vi "Detach Servo.vi"(0 "Arduino Resource":T1={"VISA resource"="", "Board Type"=enum."Arduino Uno", "Connection Type"=enum."USB / Serial", "Bytes Per Packet (15)"=15}, 5 "Servo Number":u8, 11 "error in":errorcluster) -> (4 "Arduino Resource":T1={"VISA resource"="", "Board Type"=enum."Arduino Uno", "Connection Type"=enum."USB / Serial", "Bytes Per Packet (15)"=15}, 15 "error out":errorcluster)   [LabVIEW 2011, in "LabVIEW Interface for Arduino.lvlib"]
doc: "Detach Servo release the servo from its assigned pin allowing you to use the DIO pin for general purpose digital input and output."
uses:
  <vilib>/LabVIEW Interface for Arduino/LabVIEW Interface for Arduino.lvlib
  <vilib>/LabVIEW Interface for Arduino/Private/Type Defs/Arduino Resource.ctl
  <vilib>/LabVIEW Interface for Arduino/Private/Type Defs/Board Type.ctl
  <vilib>/LabVIEW Interface for Arduino/Private/Type Defs/Command.ctl
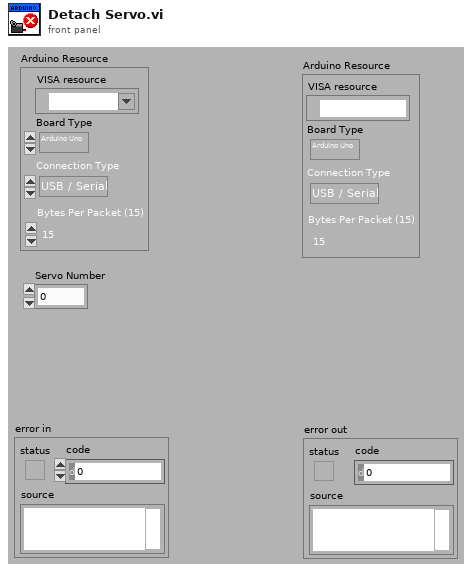
[diagram p1: front panel]
types:
  T1 = typedef "LabVIEW Interface for Arduino.lvlib/Arduino Resource.ctl" = cluster{"VISA resource":refnum<visa-resource-name>, "Board Type":T2, "Connection Type":enum8{"USB / Serial"}, "Bytes Per Packet (15)":u8}
  T2 = typedef "LabVIEW Interface for Arduino.lvlib/Board Type.ctl" = enum16{"Arduino Uno", "Dimuelanove w/Atmega 328", "Mega 2560", "Chipkit Uno32", "Chipkit Max32"}
  T3 = typedef "LabVIEW Interface for Arduino.lvlib/Command.ctl" = enum8{"setArduinoMode", "flushSerial", "setPinMode", "digitalWritePin", "digitalWritePort", "tone", "digitalReadPin", "digitalReadPort", "analogReadPin", "analogReadPort", "pwmWritePin", "pwmWritePort", "sevenSegment_Configure", "sevenSegment_Write", "I2C Init", "I2C Write", "I2C Read", "SPI Init", "SPI Set Bit Order", "SPI Set Clock Divider", "SPI Set Data Mode", "SPI Send / Receive", "SPI Close", "Servo Set Num Servos", "Servo Config Servo", "Servo Write Angle", "Servo Read Angle", "Servo Write Pulse Width", "Servo Read Pulse Width", "Servo Detach", "LCD Init", "LCD Set Size", "LCD Set Cursor Mode", "LCD Clear", "LCD Set Cursor Position", "LCD Print", "LCD Display Power", "LCD Scroll Display", "LCD Autoscroll", "LCD Print Direction", "LCD Create Custom Char", "LCD Print Custom Char", "contAcqOn", "contAcqOff", "getFirmwareVersion", "FiniteSampleStart"}
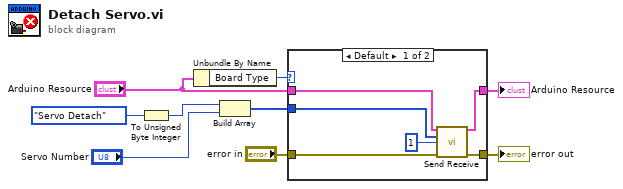
[diagram p0: block diagram]
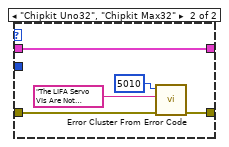
[diagram p2: hidden frame]
diagram:
  n1 = To Unsigned Byte Integer(number=Command."Servo Detach" ("Command")) -> (unsigned 8bit integer=w8:u8)
  n2 = Unbundle By Name("Arduino Resource") -> ("Board Type"=w2:T2)
  n3 = Build Array(w8, "Servo Number") -> (w6:u8[])
  n4 = case shown="Default" w2 {
    tunnel: "error in" -> [w14 w18]
    tunnel: [w11 w17] -> w4
    tunnel: "Arduino Resource" -> [w13 w16]
    tunnel: [w12 w16] -> w5
    tunnel: w6 -> [w10 _]
    frame Default {
      n5 = call <vilib>:"Send Receive.vi"("Arduino Resource"=w13, "Data"=w10, "Bytes To Read (0)"=u8 1, "error in"=w14) -> ("Arduino Resource"=w12:T1, "error out"=w11:errorcluster)  [unwired: 9 in, 1 out]
    }
    frame "Chipkit Uno32", "Chipkit Max32" {
      n6 = call <vilib>:"Error Cluster From Error Code.vi"("error in (no error)"=w18, "error message (\"\")"="The LIFA Servo VIs Are Not Supported On Chipkit Targets." ("source"), "error code (0)"=5010) -> ("error out"=w17:errorcluster)  [unwired: 6 in]
    }
  }
  "Arduino Resource" <- w5
  "error out" <- w4
